vi "FindLast.vi"(9 "pattern":string, 11 "String":string) -> (1 "after":string, 3 "before":string)   [LabVIEW 2020]
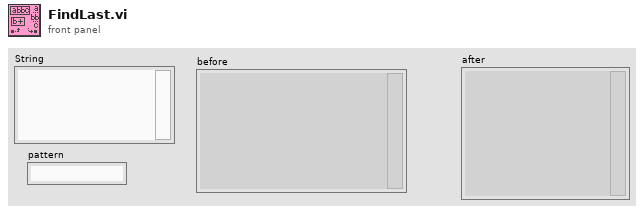
[diagram p1: front panel]
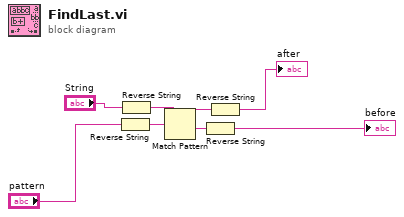
[diagram p0: block diagram]
diagram:
  n1 = Reverse String(1:"pattern") -> (0:w8:string)
  n2 = Reverse String(1:"String") -> (0:w7:string)
  n3 = Match Pattern(string=w7, regular expression=w8) -> (before substring=w3:string, after substring=w6:string)  [unwired: 1 in, 2 out]
  n4 = Reverse String(1:w6) -> (0:→"before":string)
  n5 = Reverse String(1:w3) -> (0:→"after":string)
